vi "open save dataset.vi"(9 "old dataset":T1) -> (1 "new dataset":T1)   [LabVIEW 2021]
panel:
  out "# of loaded dataset":i32
  in  "Update scale":bool=TRUE
  in  "Save dataset":bool
  in  "Open dataset":bool
  in  "Done":bool
  in  "Cancel button":bool
  # "Load or Save dataset. \nDataset includes raw data, data names, scales, show/hide indices parameters."
  # "On: Scale parameters defined by 'scaling' function will be used."
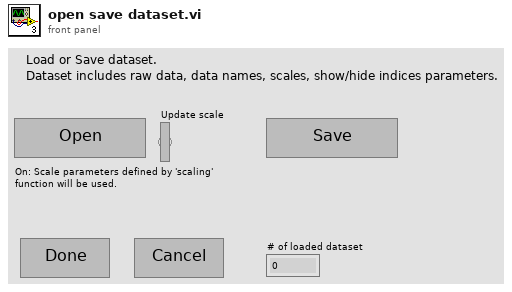
[diagram p1: front panel]
types:
  T1 = cluster{"data cluster":cluster{"all data":dbl[][]}[], "Scale":u16, "scale matrix":dbl[][], "universal y-scale":dbl, "data names":string[], "new dataset?":bool, "show files 2":cluster{"String":string, "Boolean":bool, "begin":u32, "length":u32, "y weight":dbl}[]}
  T2 = enum16{"Left Button", "Center Button", "Right Button", "Window Close"}
  T3 = cluster{"String":string, "Boolean":bool, "begin":u32, "length":u32, "y weight":dbl}[]
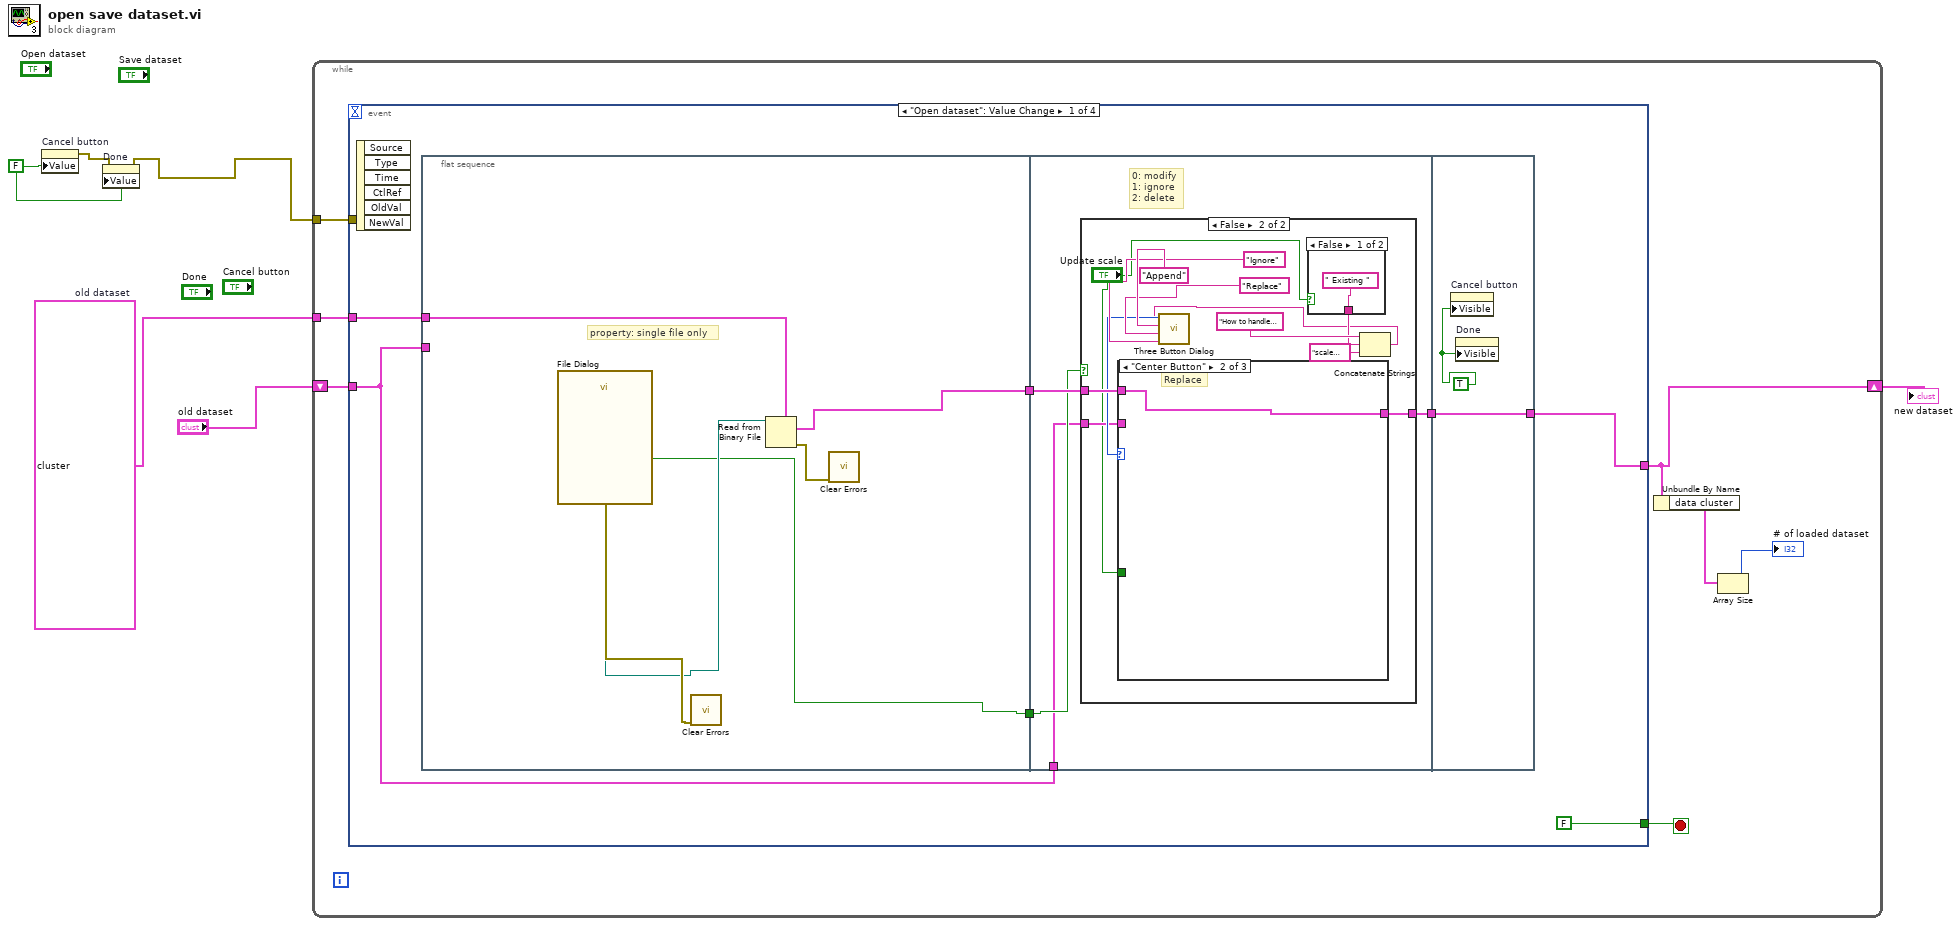
[diagram p0: block diagram]
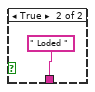
[diagram p3: hidden frame]
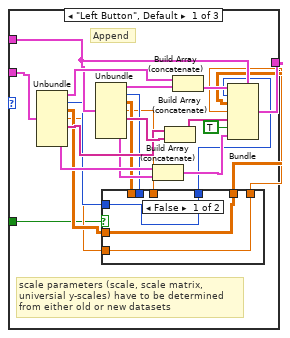
[diagram p4: hidden frame]
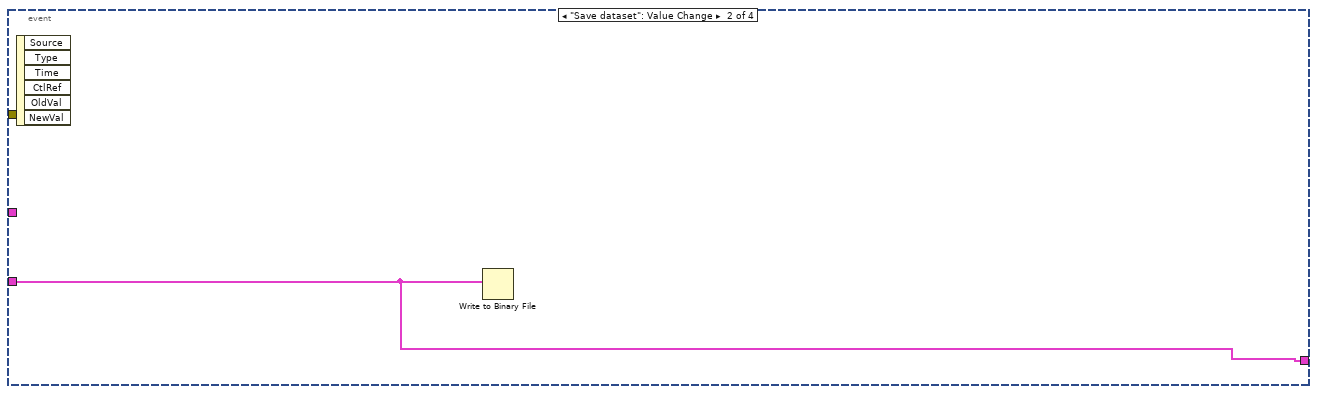
[diagram p7: hidden frame]
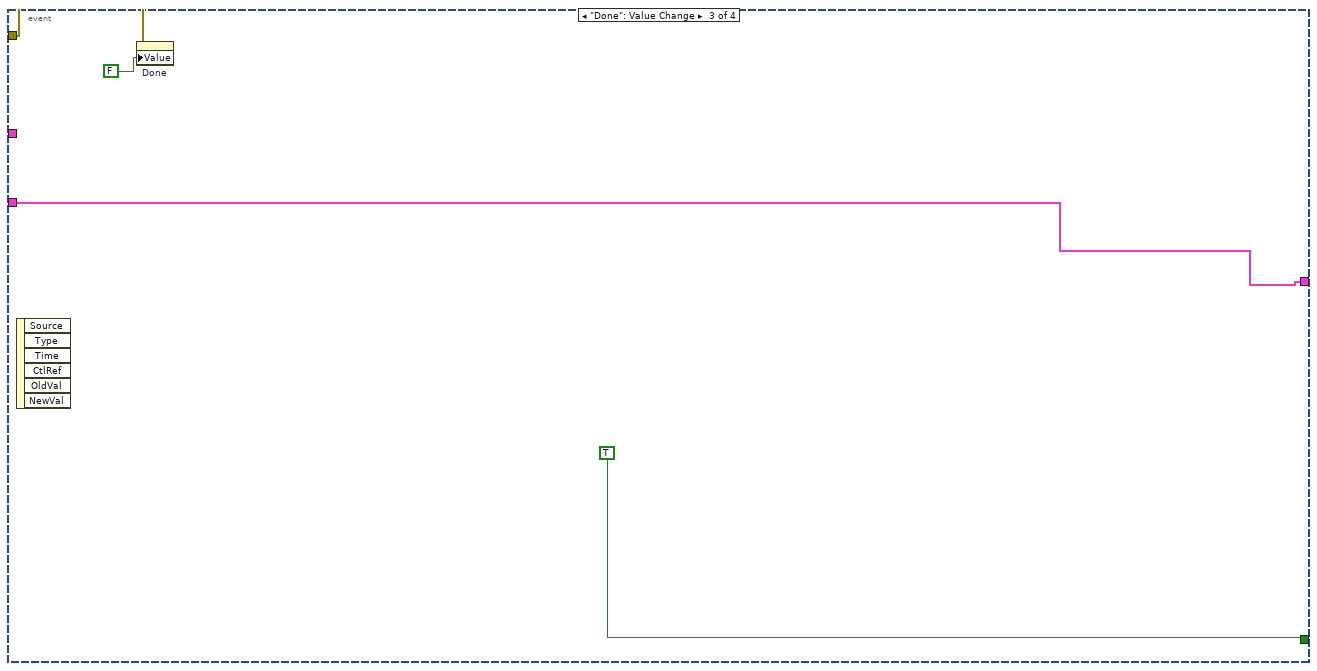
[diagram p8: hidden frame]
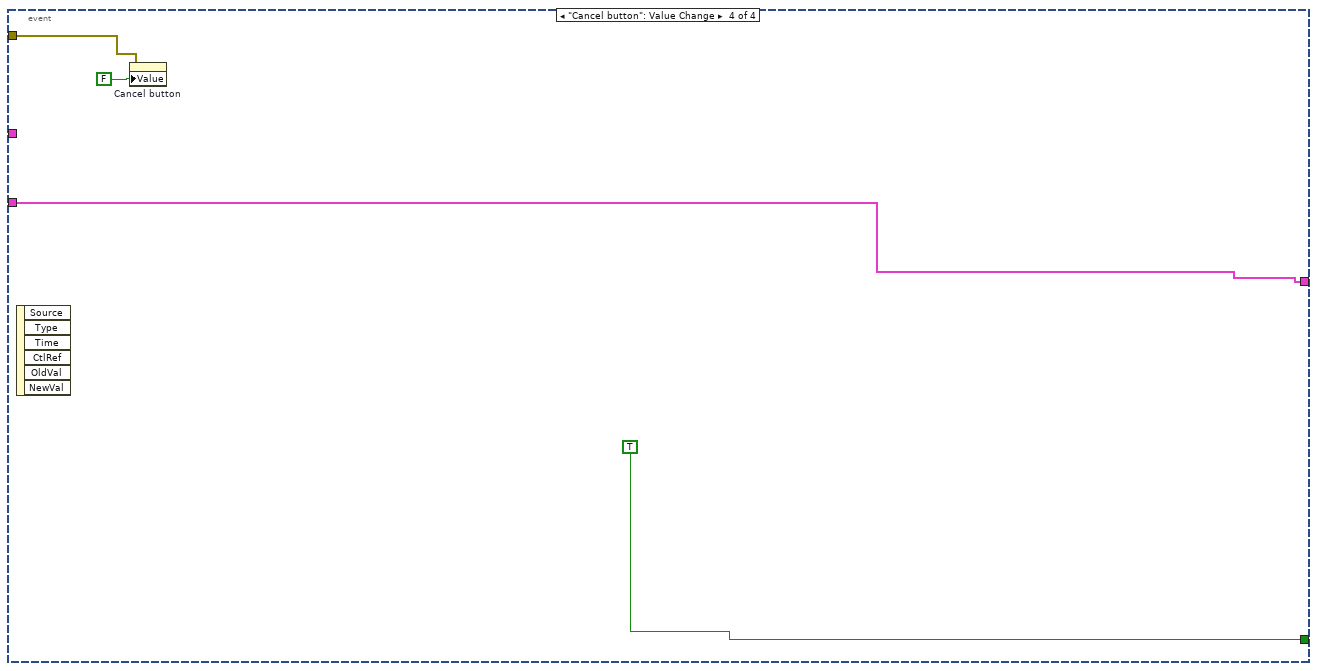
[diagram p9: hidden frame]
diagram:
  w2 = T1 {"data cluster"=[{"all data"=array60x36[2160 elements]}], "Scale"=0, "scale matrix"=[], "universal y-scale"=1.0, "data names"=["FGT512para_PPMS_Hsweep_170K3.dat"], "new dataset?"=TRUE, "show files 2"=[]}  # old dataset
  w5 = FALSE ("Value (Signaling)")
  n1 = property on="Cancel button" class="Bool (strict)"("Value"=w5) -> (error out=w6:errorcluster)  [unwired: 2 in, 1 out]
  n2 = property on="Done" class="Bool (strict)"(error in=w6, "Value"=w5) -> (error out=w4:errorcluster)  [unwired: 1 in, 1 out]
  n3 = while {
    tunnel: w4 -> [w12]
    tunnel: w2 -> [w10]
    shift-right: [w7] -> w1
    shift-left: "old dataset" -> [w11]
    stop <- w13 stop-if-true
    n4 = event shown="[0] \"Open dataset\": Value Change" {
      selector: _ -> [_ _ _ _]
      dyn-events: _ -> [_ _ _ _]
      timeout: _ -> [_ _ _ _]
      tunnel: [FALSE _ TRUE TRUE] -> w13
      tunnel: [w19 w79 w80 w84] -> w7
      tunnel: w12 -> [_ _ w82 w86]
      tunnel: w11 -> [w15 w79 w80 w84]
      tunnel: w10 -> [w14 _ _ _]
      event "Open dataset": Value Change {
        n5 = event-data() -> ()  [unwired: 1 in, 6 out]
        n6 = flat-sequence {
          tunnel: [w23] -> w18
          tunnel: [w24] -> w16
          tunnel: w15 -> [_]
          tunnel: w14 -> [w22]
          tunnel: w18 -> [w30]
          tunnel: w15 -> [w27]
          tunnel: [w29] -> w17
          tunnel: w16 -> [w28]
          tunnel: [w78] -> w19
          tunnel: w17 -> [w78]
          frame #0 {
            # "property: single file only"
            n7 = call "File Dialog"() -> ("selected path"=w25:path, "cancelled"=w24:bool, "error out"=w26:errorcluster)  [unwired: 12 in, 1 out]
            n8 = call <vilib>:"Clear Errors.vi"("error in (no error)"=w26) -> ()  [unwired: 5 in, 2 out]
            n9 = Read from Binary File(5:w22, 11:w25) -> (0:w21:errorcluster, 2:w23:T1)  [unwired: 4 in, 2 out]
            n10 = call <vilib>:"Clear Errors.vi"("error in (no error)"=w21) -> ()  [unwired: 5 in, 2 out]
          }
          frame #1 {
            # "0: modify\n1: ignore\n2: delete"
            n11 = case shown="False" w28 {
              tunnel: w30 -> [_ w40]
              tunnel: [w31 w39] -> w29
              tunnel: w27 -> [w31 w37]
              frame True {
              }
              frame False {
                n12 = case shown="False" "Update scale" {
                  tunnel: [" Existing " ("Center Button Text (\"No\")") " Loded " ("Center Button Text (\"No\")")] -> w34
                  frame False {
                  }
                  frame True {
                  }
                }
                n13 = Concatenate Strings("How to handle the loaded dataset?" ("message"), w34, "scale parameters will be used." ("string")) -> (w32:string)
                n14 = call <vilib>:"Three Button Dialog.vi"("Right Button Text (\"Cancel\")"="Ignore" ("Right Button Text (\"Cancel\")"), "Center Button Text (\"No\")"="Replace" ("Center Button Text (\"No\")"), "Left Button Text (\"Yes\")"="Append" ("Left Button Text (\"Yes\")"), "message"=w32) -> ("Which Button?"=w38:T2)  [unwired: 7 in]
                n15 = case shown="\"Center Button\"" w38 {
                  tunnel: [w57 w75 w76] -> w39
                  tunnel: w40 -> [w61 w75 _]
                  tunnel: w37 -> [w68 _ w76]
                  tunnel: "Update scale" -> [w46 _ _]
                  frame "Left Button", Default {
                    # "scale parameters (scale, scale matrix, \nuniversial y-scales) have to be determined\nfrom either old or new datasets"
                    # "Append"
                    n16 = Unbundle(w68) -> ("data cluster"=w67:cluster{"all data":dbl[][]}[], "Scale"=w49:u16, "scale matrix"=w48:dbl[][], "universal y-scale"=w47:dbl, "data names"=w63:string[], "show files 2"=w59:T3)  [unwired: 1 out]
                    n17 = Unbundle(w61) -> ("data cluster"=w66:cluster{"all data":dbl[][]}[], "Scale"=w54:u16, "scale matrix"=w52:dbl[][], "universal y-scale"=w50:dbl, "data names"=w64:string[], "show files 2"=w58:T3)  [unwired: 1 out]
                    n18 = case shown="False" w46 {
                      tunnel: [w71 w74] -> w55
                      tunnel: w54 -> [_ w74]
                      tunnel: [w70 w73] -> w53
                      tunnel: w52 -> [_ w73]
                      tunnel: [w69 w72] -> w51
                      tunnel: w50 -> [_ w72]
                      tunnel: w49 -> [w71 _]
                      tunnel: w48 -> [w70 _]
                      tunnel: w47 -> [w69 _]
                      frame False {
                      }
                      frame True {
                      }
                    }
                    n19 = Build Array (concatenate)(w59, w58) -> (w56:T3)
                    n20 = Build Array (concatenate)(w63, w64) -> (w62:string[])
                    n21 = Build Array (concatenate)(w67, w66) -> (w65:cluster{"all data":dbl[][]}[])
                    n22 = Bundle(cluster=w61, "data cluster"=w65, "Scale"=w55, "scale matrix"=w53, "universal y-scale"=w51, "data names"=w62, "new dataset?"=TRUE, "show files 2"=w56) -> (w57:T1)
                  }
                  frame "Center Button" {
                    # "Replace"
                  }
                  frame "Right Button" {
                    # "Ignore"
                  }
                }
              }
            }
          }
          frame #2 {
            w77 = TRUE ("Visible")
            n23 = property on="Cancel button" class="Bool (strict)"("Visible"=w77) -> ()  [unwired: 2 in, 2 out]
            n24 = property on="Done" class="Bool (strict)"("Visible"=w77) -> ()  [unwired: 2 in, 2 out]
          }
        }
      }
      event "Save dataset": Value Change {
        n25 = event-data() -> ()  [unwired: 1 in, 6 out]
        n26 = Write to Binary File(data=w79) -> ()  [unwired: 5 in, 3 out]
      }
      event "Done": Value Change {
        n27 = event-data() -> ()  [unwired: 1 in, 6 out]
        n28 = property on="Done" class="Bool (strict)"(error in=w82, "Value"=FALSE ("Value (Signaling)")) -> ()  [unwired: 1 in, 2 out]
      }
      event "Cancel button": Value Change {
        n29 = event-data() -> ()  [unwired: 1 in, 6 out]
        n30 = property on="Cancel button" class="Bool (strict)"(error in=w86, "Value"=FALSE ("Value (Signaling)")) -> ()  [unwired: 1 in, 2 out]
      }
    }
    n31 = Unbundle By Name(w7) -> ("data cluster"=w8:cluster{"all data":dbl[][]}[])
    n32 = Array Size(array=w8) -> (size(s)=→"# of loaded dataset":i32)
  }
  "new dataset" <- w1
